vi "LVClass_ModalCoef SetData.vi"(0 "ModalCoef in":refnum<class "ModalCoef.lvclass">, 5 "coef":sgl[](array[numeric]), 7 "index":u32[](array[numeric]), 9 "Pupil.lvclass":refnum<class "Pupil.lvclass">, 11 "error in (no error)":errorcluster) -> (4 "ModalCoef out":refnum<class "ModalCoef.lvclass">, 8 "index":u32[](array[numeric]), 10 "Pupil (dup)":refnum<class "Pupil.lvclass">, 15 "error out":errorcluster)   [LabVIEW 2020, in "ModalCoef.lvclass"]
doc: "Set polynomial coefficients informations and values.\n\n--------------------------------------------------------------------------------\n\n<B>TypePhaseIn </B> : TypePhase phase mode reconstruction.\n<B>TypePhaseOut </B> : TypePhase phase mode reconstruction.\n<B>modalCoef </B> : ModalCoef object.\n<B>coef </B> : Array of modal coefficient values.\n<B>index </B> : Array of modal coefficient indices.\n<B>size </B> : Size of the coefficient array.\n<B>pupil </B> : pupil object.\n<B>ErrorIn </B> : Error\n<B>ErrorOut </B> : Error\n\n--------------------------------------------------------------------------------"
uses:
  ModalCoef.lvclass
  Pupil.lvclass
  ModalCoef.lvclass/ModalCoef.ctl
  LVClass_Pupil Read Pupil.vi
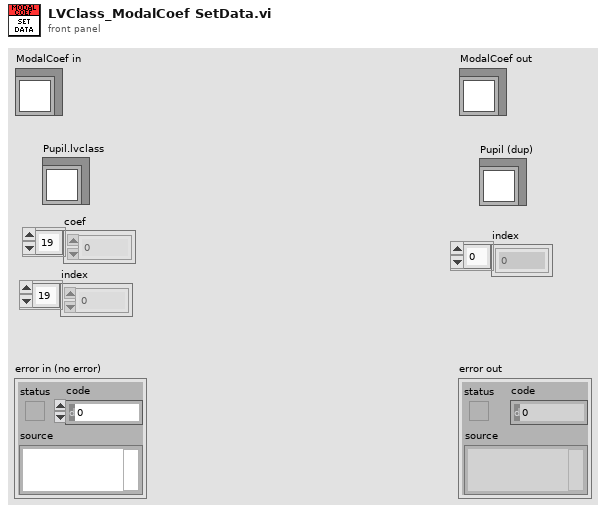
[diagram p1: front panel]
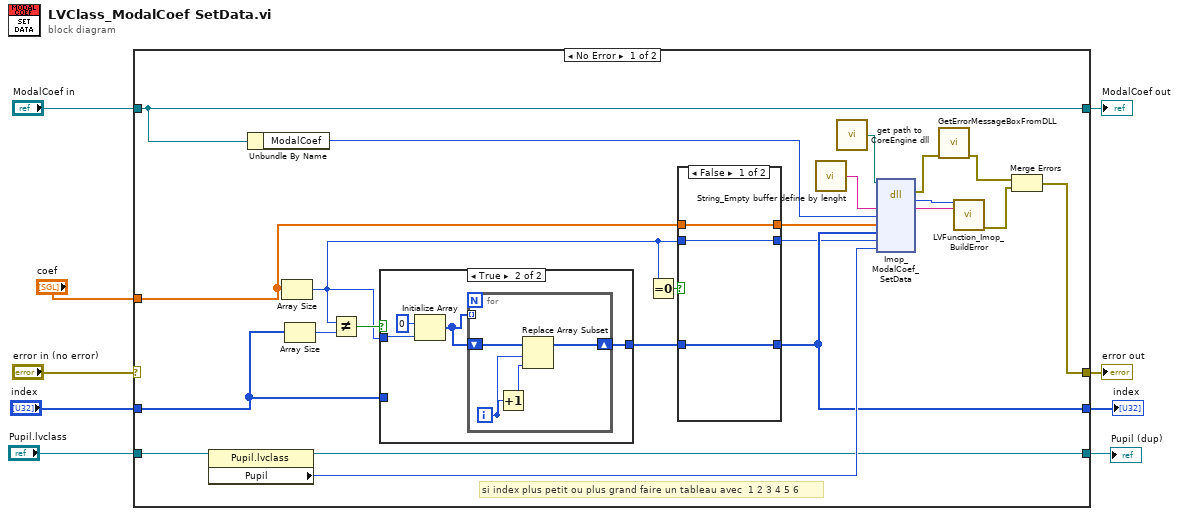
[diagram p0: block diagram]
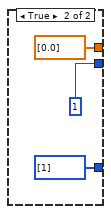
[diagram p2: hidden frame]
diagram:
  n1 = case shown="No Error" "error in (no error)" {
    selector: "error in (no error)" -> [_ w51]
    tunnel: [w19 w51] -> w8
    tunnel: [w26 w50] -> w6
    tunnel: "ModalCoef in" -> [w26 w50]
    tunnel: "Pupil.lvclass" -> [w25 w48]
    tunnel: [w12 w49] -> w4
    tunnel: "index" -> [w18 w49]
    tunnel: [w17 w48] -> w2
    tunnel: "coef" -> [w14 _]
    frame No Error {
      # "si index plus petit ou plus grand faire un tableau avec  1 2 3 4 5 6"
      n2 = property class="Pupil.lvclass"(reference=w25) -> (reference out=w17:refnum<class "Pupil.lvclass">, "Pupil"=w24:i32)  [unwired: 1 in, 1 out]
      n3 = Unbundle By Name(w26) -> ("ModalCoef"=w27:i32)
      n4 = Array Size(array=w14) -> (size(s)=w10:i32)
      n5 = Array Size(array=w18) -> (size(s)=w23:i32)
      n6 = Not Equal?(x=w10, y=w23) -> (x != y?=w22:bool)
      n7 = case shown="True" w22 {
        tunnel: w10 -> [_ w41]
        tunnel: w18 -> [w39 _]
        tunnel: [w39 w40] -> w16
        frame False {
        }
        frame True {
          n8 = Initialize Array(u32 0, w41) -> (w42:u32[])
          n9 = for {
            shift-right: [w44] -> w40
            shift-left: w42 -> [w45]
            tunnel: w42 -> [_] mode=indexing
            i -> [w46]
            n10 = Increment(x=w46) -> (x+1=w47:i32)
            n11 = Replace Array Subset(array=w45, new element=w47, index=w46) -> (w44:u32[])
          }
        }
      }
      n12 = Equal To 0?(x=w10) -> (x = 0?=w15:bool)
      n13 = case shown="False" w15 {
        tunnel: w16 -> [w34 _]
        tunnel: w14 -> [w35 _]
        tunnel: [w35 sgl[] [0.0] ("coef")] -> w13
        tunnel: [w34 u32[] [1] ("index")] -> w12
        tunnel: [w33 u32 1] -> w11
        tunnel: w10 -> [w33 _]
        frame False {
        }
        frame True {
        }
      }
      n14 = call "String_Empty buffer define by lenght.vi"() -> ("Empty buffer"=w32:string)  [unwired: 1 in]
      n15 = call "get path to CoreEngine dll.vi"() -> ("path to c_interface_vc100.dll"=w29:path)  [unwired: 12 in, 3 out]
      n16 = dll-call lib="D:/2_trunk/Soft_haso/ImOpCoreEngine4_LV2011/DLLs/ImopEngine4_vc100.dll" fn="Imop_ModalCoef_SetData"(path in=w29, "message"=w32, "ModalCoefs"=w27, "coef"=w13, "index"=w12, "size"=w11, "pupil"=w24) -> (error out=w28:errorcluster, "return type"=w30:i32, "message"=w31:string)  [unwired: 7 in, 1 out]
      n17 = call "GetErrorMessageBoxFromDLL.vi"("error IN"=w28) -> ("error OUT"=w21:errorcluster)  [unwired: 10 in]
      n18 = call "LVFunction_Imop_BuildError.vi"("code"=w30, "String to Prepend to source (\"\")"=w31) -> ("error out"=w20:errorcluster)  [unwired: 13 in]
      n19 = Merge Errors(w21, w20) -> (w19:errorcluster)
    }
    frame Error {
    }
  }
  "error out" <- w8
  "ModalCoef out" <- w6
  "Pupil (dup)" <- w2
  "index" <- w4
